vi "Pattern Matching.vi"() -> ()   [LabVIEW 2018]
uses:
  <vilib>/vision/NI_Vision_Development_Module.lvlib
panel:
  out "# of Matches":i32
  in  "Stop Button":bool
  out "Calibrated":bool
  out "Template":T1(plugin-control)
  out "Matches (pixel)":T2(array[cluster])
  in  "Settings":T3={"Algorithm"=enum."Low Discrepancy Sampling", "Number of Matches Requested"=1, "Minimum Match Score"=0.0, "SubPixel Accuracy"=TRUE, "Rotation Angles Ranges"=[{"Start"=0.0, "End"=0.0}], "Show Search Area"=FALSE, "Show Result"=TRUE} {"Minimum Match Score" min=0 max=1000 format="%.2f"; "Number of Matches Requested" min=1}
  in  "Pattern":T4(ring)
  out "Camera Image":T1(plugin-control)
  # "Mechatronic Systems Board"
  # "Pattern Matching"
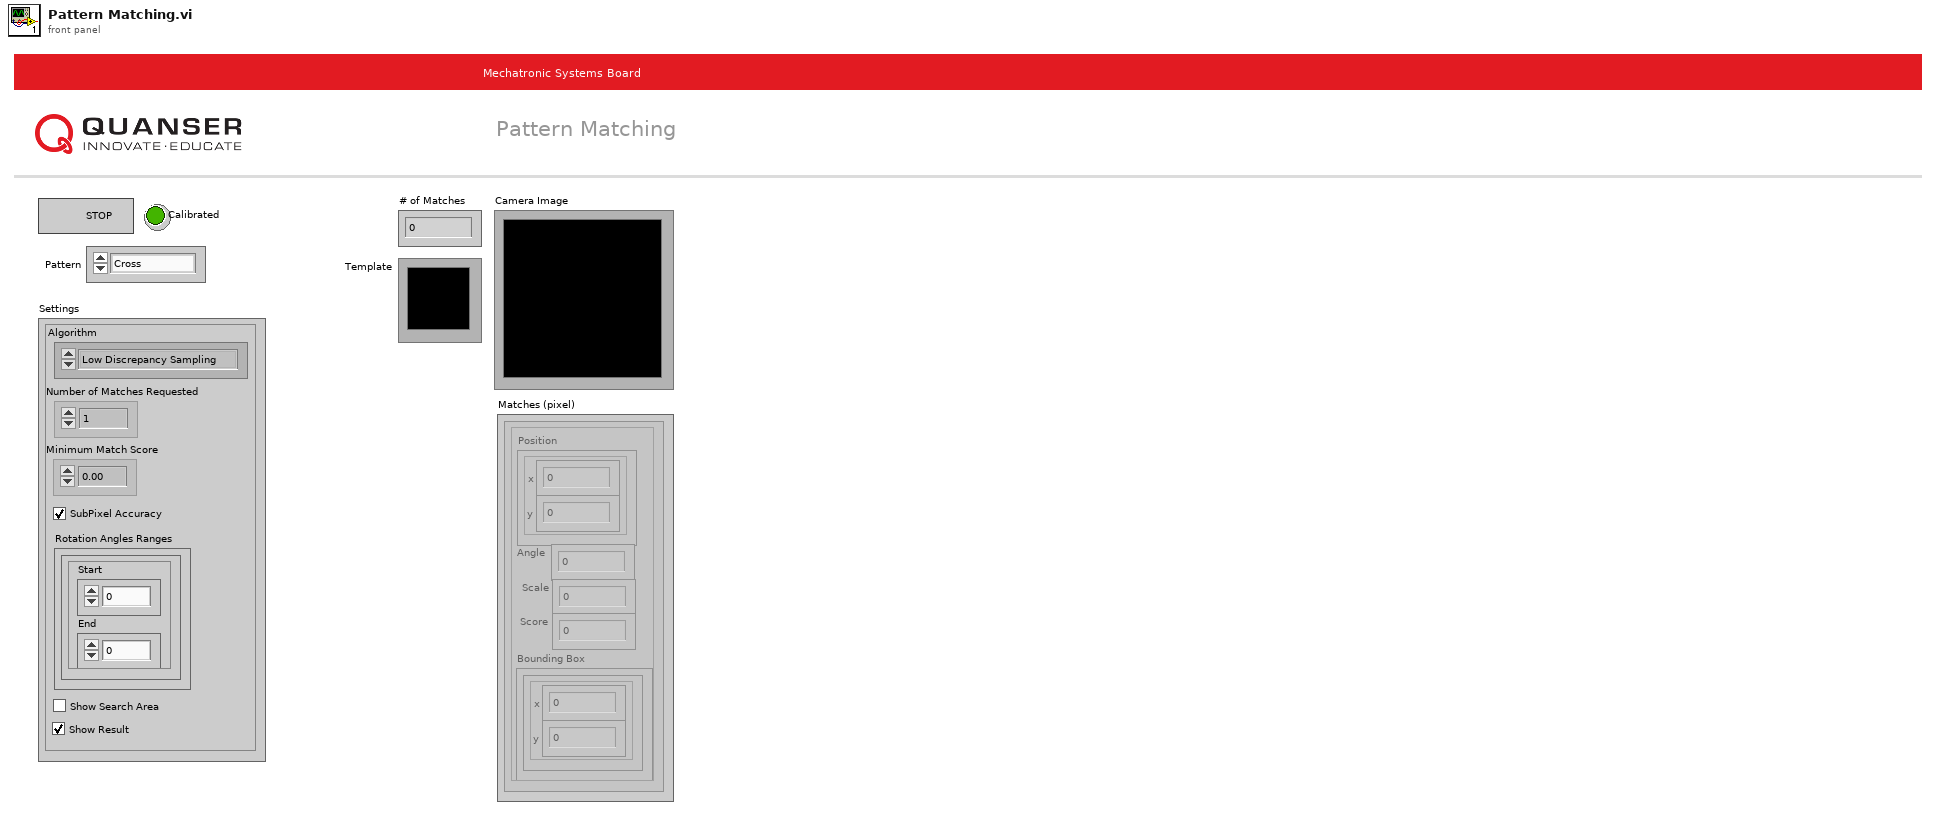
[diagram p1: front panel]
types:
  T1 = typedef "IMAQ Image.ctl" = refnum<image>
  T2 = cluster{"Position":cluster{"x":dbl, "y":dbl}, "Angle":dbl, "Scale":dbl, "Score":dbl, "Bounding Box":cluster{"x":dbl, "y":dbl}[]}[]
  T3 = cluster{"Algorithm":enum16{"All", "Low Discrepancy Sampling", "Grayscale Value Pyramid", "Gradients Pyramid"}, "Number of Matches Requested":i32, "Minimum Match Score":sgl, "SubPixel Accuracy":bool, "Rotation Angles Ranges":cluster{"Start":dbl, "End":dbl}[], "Show Search Area":bool, "Show Result":bool}
  T4 = enum16{"Cross", "Police", "Fire", "Library", "School", "Airport", "North", "Branch"}
  T5 = typedef "QNET MS IO Cluster.ctl" = cluster{"Error":errorcluster, "Encoder Calibration Values":i32[], "Update Calibration":bool, "JPEG Resolutions":u16, "Raw Resolutions":u16, "Image Mode":enum16{"RAW RGB", "RAW Gray Scale", "JPEG"}, "FPGA Ref":refnum<k20>}
  T6 = cluster{"Position":cluster{"x":sgl, "y":sgl}, "Angle":sgl, "Scale":sgl, "Score":sgl, "Bounding Box":cluster{"x":sgl, "y":sgl}[]}[]
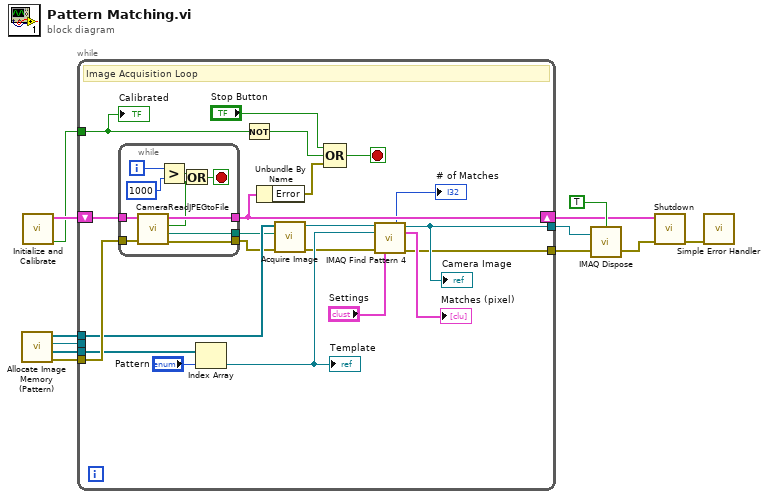
[diagram p0: block diagram]
diagram:
  n1 = call "Allocate Image Memory (Pattern).vi"() -> ("error out"=w8:errorcluster, "Template Patterns"=w5:T1[], "Process Memory"=w4:T1, "Acquisition Memory"=w6:T1[])  [unwired: 8 in]
  n2 = call "Initialize and Calibrate.vi"() -> ("Calibrated"=w3:bool, "IO Cluster"=w7:T5)  [unwired: 10 in]
  n3 = while {
    tunnel: [w20] -> w11
    tunnel: [w25] -> w10
    tunnel: w8 -> [w31]
    tunnel: w6 -> [w30]
    tunnel: w5 -> [w29]
    tunnel: w4 -> [_]
    tunnel: w3 -> [w19]
    shift-right: [w16] -> w2
    shift-left: w7 -> [w32]
    stop <- w14 stop-if-true
    # "Image Acquisition Loop"
    n4 = while {
      tunnel: [w39] -> w28
      tunnel: w32 -> [w43]
      tunnel: [w42] -> w16
      tunnel: w31 -> [w40]
      tunnel: [w41] -> w22
      i -> [w35]
      stop <- w38 stop-if-true
      n5 = call "CameraReadJPEGtoFile.vi"("error in"=w40, "IO Cluster In"=w43) -> ("Error Out"=w41:errorcluster, "Image File"=w39:path, "New Image Data"=w34:bool, "IO Cluster Out"=w42:T5)  [unwired: 6 in]
      n6 = Greater?(x=w35, y=1000) -> (0:w37:bool)
      n7 = Or(x=w37, y=w34) -> (x .or. y?=w38:bool)
    }
    n8 = Index Array(array=w29, index="Pattern") -> (element=w26:T1)
    "Template" <- w26
    n9 = Not(x=w19) -> (.not. x?=w17:bool)
    n10 = Unbundle By Name(w16) -> ("Error"=w15:errorcluster)
    n11 = call "Acquire Image.vi"("Error In"=w22, "File Path"=w28, "Acquisition Memory"=w30) -> ("Error Out"=w21:errorcluster, "Pre-processed Image"=w27:T1)  [unwired: 4 in, 3 out]
    n12 = Compound Arithmetic op=OR("Stop Button", w17, w15) -> (w14:bool)
    n13 = call "IMAQ Find Pattern 4"("Image"=w27, "Template"=w26, "error in"=w21, "Settings"="Settings") -> ("Number of Matches"=→"# of Matches":i32, "Image Out"=w25:T1, "Matches (pixel)"=→"Matches (pixel)":T6, "error out"=w20:errorcluster)  [unwired: 5 in, 3 out]
    "Camera Image" <- w25
    "Calibrated" <- w19
  }
  n14 = call "IMAQ Dispose"("All Images? (No)"=TRUE, "Image"=w10, "error in (no error)"=w11) -> ("error out"=w12:errorcluster)  [unwired: 3 in]
  n15 = call "Shutdown.vi"("Image Processing Loop"=w12, "IO Cluster In"=w2) -> ("Error"=w1:errorcluster)  [unwired: 9 in]
  n16 = call <vilib>:"Simple Error Handler.vi"("error in (no error)"=w1) -> ()  [unwired: 4 in, 5 out]
